vi "SM User Interface.vi"() -> ()   [LabVIEW 2021]
panel:
  in  "C":bool
  in  "B":bool
  in  "A":bool
  out "State 3":bool
  out "State 2":bool
  out "State 1":bool
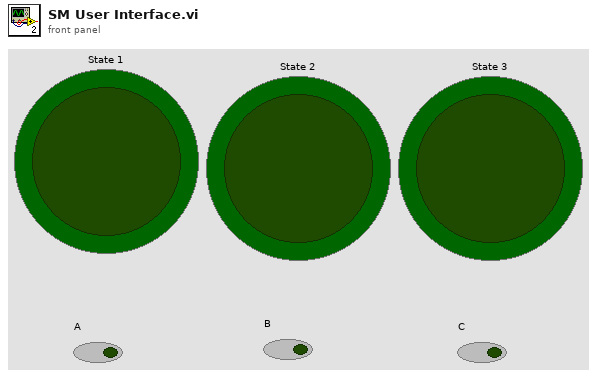
[diagram p1: front panel]
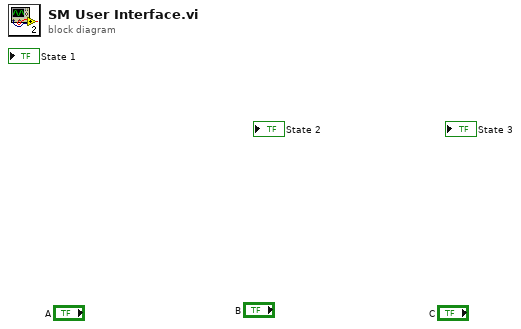
[diagram p0: block diagram]
diagram:
